vi "PicoScope3000aGetRapidBlockBulk.vi"(0 "error in":errorcluster, 5 "Number of Segments":u32, 7 "handle in":i16, 9 "Device Info":T1, 11 "Rapid Block Bulk Acquisition Settings":T2 {"Down Sample Ratio" min=1 step=1; "Down-Sample Mode" items=["None", "Aggregate", "Decimate", "Average"]}) -> (2 "Channel A Buffer":i16[][](array[numeric]), 3 "Channel B Buffer":i16[][](array[numeric]), 4 "error out":errorcluster, 6 "handle out":i16, 10 "Port 0 Buffer":i16[][](array[numeric]), 12 "Num samples":u32, 13 "Channel C Buffer":i16[][](array[numeric]), 14 "Channel D Buffer":i16[][](array[numeric]), 15 "Port 1 Buffer":i16[][](array[numeric]))   [LabVIEW 2009]
doc: "This VI gets a set of blocks captured using rapid block mode. It outputs two-dimensional arrays for each channel that contain data from all the requested captures."
uses:
  ps3000a.dll
panel:
  out "overflow":i16[](array[numeric])
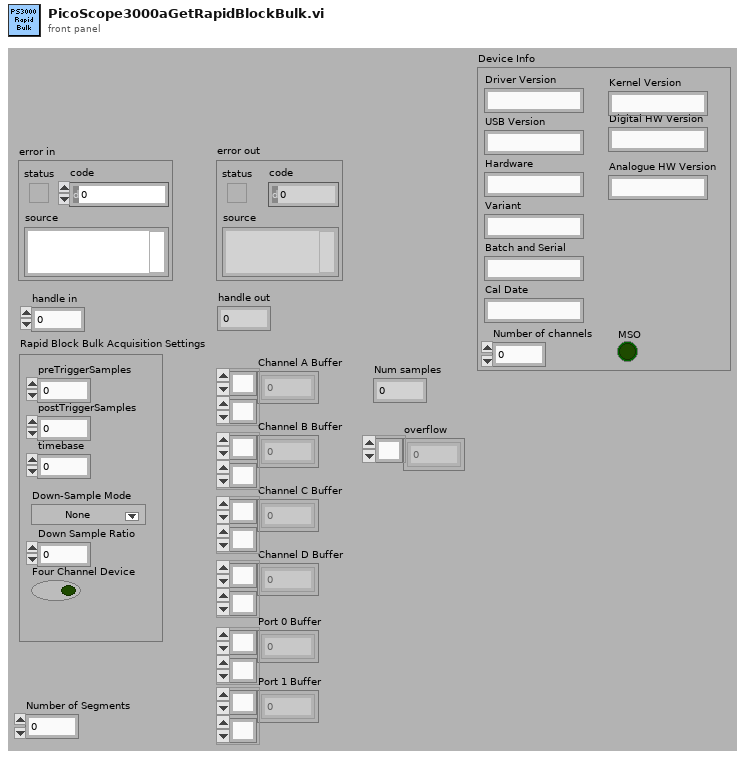
[diagram p1: front panel]
types:
  T1 = cluster{"Driver Version":string, "USB Version":string, "Hardware":string, "Variant":string, "Batch and Serial":string, "Cal Date":string, "Kernel Version":string, "Digital HW Version":string, "Analogue HW Version":string, "MSO":bool, "Number of channels":i16}
  T2 = cluster{"preTriggerSamples":u32, "postTriggerSamples":u32, "timebase":u32, "Down-Sample Mode":i32, "Down Sample Ratio":u32, "Four Channel Device":bool}
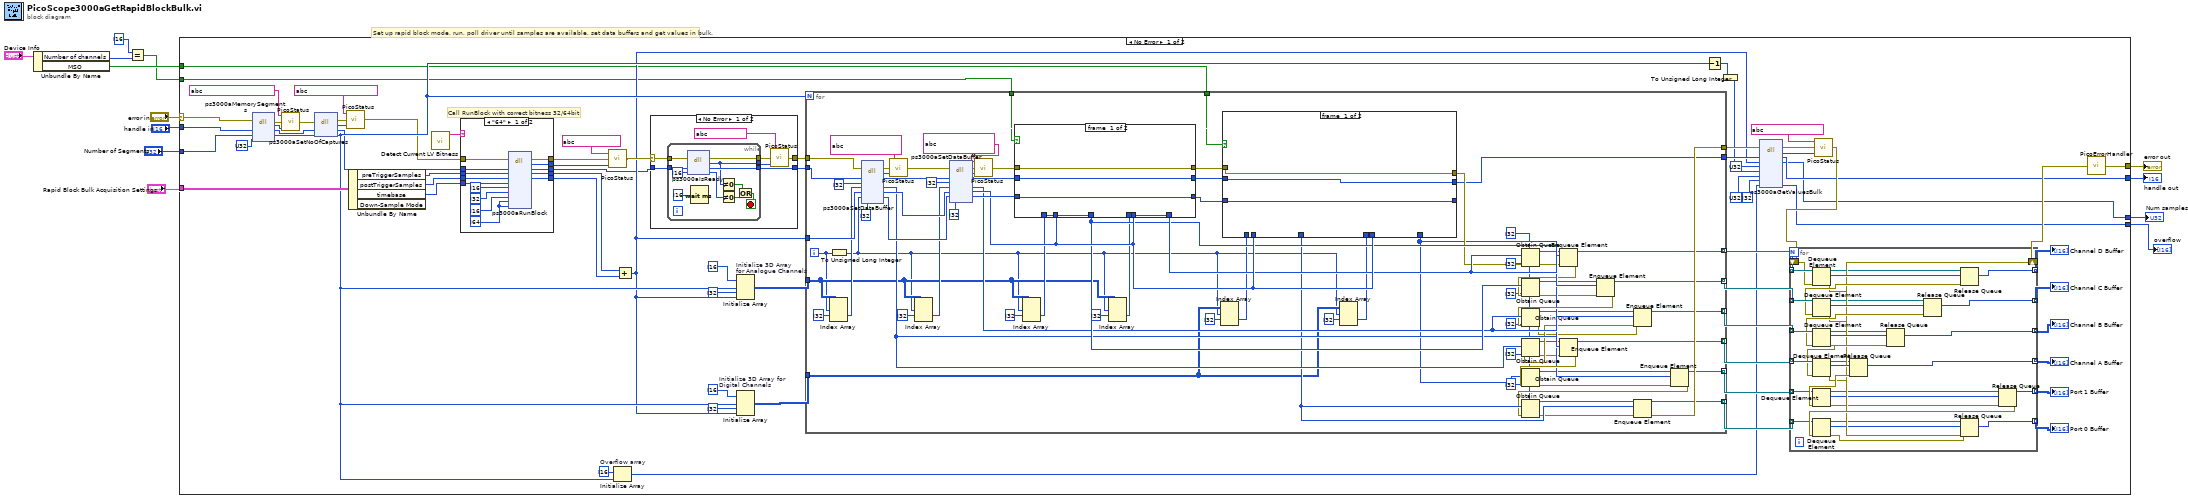
[diagram p0: block diagram]
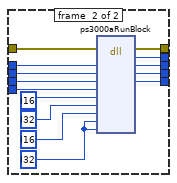
[diagram p2: hidden frame]
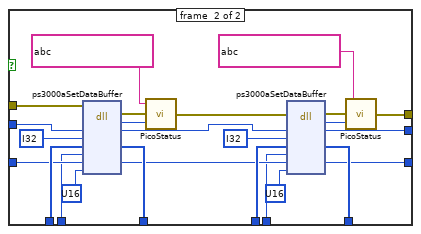
[diagram p3: hidden frame]
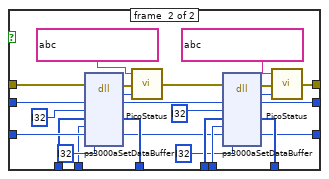
[diagram p4: hidden frame]
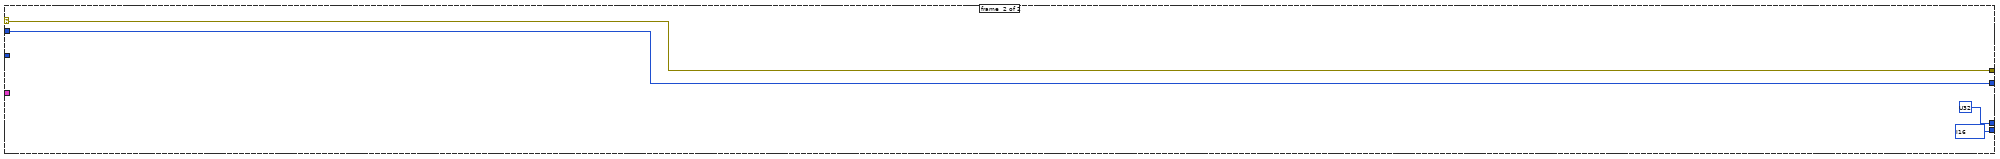
[diagram p6: hidden frame]
diagram:
  # "Set up rapid block mode, run, poll driver until samples are available, set data buffers and get values in bulk."
  n1 = Unbundle By Name("Device Info") -> ("Number of channels"=w4:i16, "MSO"=w5:bool)
  n2 = Equal?(x=i16 ?, y=w4) -> (x = y?=w2:bool)
  n3 = case shown="No Error" "error in" {
    selector: "error in" -> [w78 w303]
    tunnel: [w66 w303] -> w12
    tunnel: "handle in" -> [w77 w302]
    tunnel: [w56 w302] -> w10
    tunnel: [w31 u32 ?] -> w9
    tunnel: "Rapid Block Bulk Acquisition Settings" -> [w29 _]
    tunnel: "Number of Segments" -> [w28 _]
    tunnel: w2 -> [w26 _]
    tunnel: w5 -> [w27 _]
    tunnel: [w14 i16[] ? ("overflow")] -> w1
    frame #0 {
      # "Call RunBlock with correct bitness 32/64bit"
      n4 = dll-call lib="ps3000a.dll" fn="ps3000aMemorySegments" ("ps3000.dll:_ps3000_open_unit@0")(error in=w78, "handle"=w77, "nSegments"=w28, "nMaxSamples"=u32 ?) -> (error out=w75:errorcluster, "PICO_STATUS"=w76:i32, "handle"=w71:i16, "nSegments"=w72:u32)  [unwired: 3 in, 1 out]
      n5 = call "PicoStatus.vi"("PICO STATUS"=w76, "error in"=w75, "source"=string ?) -> ("error out"=w70:errorcluster)
      n6 = dll-call lib="ps3000a.dll" fn="ps3000aSetNoOfCaptures" ("ps3000.dll:_ps3000_open_unit@0")(error in=w70, "handle"=w71, "nCaptures"=w72) -> (error out=w68:errorcluster, "PICO_STATUS"=w69:i32, "handle"=w19:i16, "nCaptures"=w34:u32)  [unwired: 2 in, 1 out]
      n7 = call "PicoStatus.vi"("PICO STATUS"=w69, "error in"=w68, "source"=string ?) -> ("error out"=w15:errorcluster)
      n8 = Unbundle By Name(w29) -> ("preTriggerSamples"=w18:u32, "postTriggerSamples"=w17:u32, "timebase"=w16:u32)  [unwired: 1 out]
      n9 = call "Detect Current LV Bitness.vi"() -> ("bitness"=w25:string)  [unwired: 11 in]
      n10 = case shown="\"64\"" w25 {
        tunnel: [w96 w110] -> w22
        tunnel: [w95 w109] -> w21
        tunnel: [w94 w108] -> w20
        tunnel: w16 -> [w93 w107]
        tunnel: w18 -> [w92 w106]
        tunnel: w17 -> [w91 w105]
        tunnel: [w90 w104] -> w23
        tunnel: [w89 w103] -> w24
        tunnel: w15 -> [w88 w102]
        tunnel: w19 -> [w87 w101]
        frame #0 {
          w83 = i64 ? ("pParameter")
          n11 = dll-call lib="ps3000a.dll" fn="ps3000aRunBlock" ("ps3000.dll:_ps3000_open_unit@0")(error in=w88, "handle"=w87, "preTriggerSamples"=w92, "postTriggerSamples"=w91, "timebase"=w93, "oversample"=i16 ?, "timeindisposed"=i32 ? ("pParameter"), "segmentIndex"=i16 ? ("pParameter"), "lpReady"=w83, "pParameter"=w83) -> (error out=w89:errorcluster, "PICO_STATUS"=w90:i32, "handle"=w96:i16, "preTriggerSamples"=w95:u32, "postTriggerSamples"=w94:u32)  [unwired: 8 in, 1 out]
        }
        frame #1 {
          w97 = i32 ? ("pParameter")
          n12 = dll-call lib="ps3000a.dll" fn="ps3000aRunBlock" ("ps3000.dll:_ps3000_open_unit@0")(error in=w102, "handle"=w101, "preTriggerSamples"=w106, "postTriggerSamples"=w105, "timebase"=w107, "oversample"=i16 ?, "timeindisposed"=i32 ? ("pParameter"), "segmentIndex"=i16 ? ("pParameter"), "lpReady"=w97, "pParameter"=w97) -> (error out=w103:errorcluster, "PICO_STATUS"=w104:i32, "handle"=w110:i16, "preTriggerSamples"=w109:u32, "postTriggerSamples"=w108:u32)  [unwired: 8 in, 1 out]
        }
      }
      n13 = call "PicoStatus.vi"("PICO STATUS"=w23, "error in"=w24, "source"=string ?) -> ("error out"=w80:errorcluster)
      n14 = Initialize Array "Overflow array"(i16 ? ("element"), w34) -> (w40:i16[])
      n15 = Add(x=w21, y=w20) -> (x+y=w33:u32)
      n16 = case shown="No Error" w80 {
        selector: w80 -> [w284 w298]
        tunnel: w22 -> [w286 w299]
        tunnel: [w285 w299] -> w82
        tunnel: [w283 w298] -> w81
        frame #0 {
          n17 = while {
            tunnel: [w297] -> w285
            tunnel: w286 -> [w296]
            tunnel: [w291] -> w281
            tunnel: w284 -> [w290]
            tunnel: [w289] -> w282
            stop <- w295 stop-if-true
            n18 = dll-call lib="ps3000a.dll" fn="ps3000aIsReady" ("ps3000.dll:_ps3000_open_unit@0")(error in=w290, "handle"=w296, "ready"=i16 ?) -> (error out=w289:errorcluster, "status"=w291:i32, "handle"=w297:i16, "ready"=w292:i16)  [unwired: 2 in, 1 out]
            n19 = Wait (ms)(milliseconds to wait=i16 ? ("ready")) -> ()  [unwired: 1 out]
            n20 = Not Equal To 0?(x=w291) -> (x != 0?=w293:bool)
            n21 = Not Equal To 0?(x=w292) -> (x != 0?=w294:bool)
            n22 = Or(x=w293, y=w294) -> (x .or. y?=w295:bool)
          }
          n23 = call "PicoStatus.vi"("PICO STATUS"=w281, "error in"=w282, "source"=string ?) -> ("error out"=w283:errorcluster)
        }
        frame #1 {
        }
      }
      n24 = Initialize Array "Initialize 3D Array\nfor Analogue Channels"(i16 ? ("element"), w34, i32 ? ("dimension size"), w33) -> (w37:i16[][][])
      n25 = Initialize Array "Initialize 3D Array for \nDigital Channels"(i16 ? ("element"), w34, i32 ? ("dimension size"), w33) -> (w32:i16[][][])
      n26 = for {
        N: w34 -> [_]
        tunnel: w82 -> [w221]
        tunnel: w81 -> [w219]
        tunnel: w26 -> [w213]
        tunnel: w27 -> [w201]
        tunnel: [w185] -> w55
        tunnel: [w184] -> w54 mode=indexing
        tunnel: [w183] -> w53 mode=indexing
        tunnel: [w182] -> w52 mode=indexing
        tunnel: [w181] -> w51 mode=indexing
        tunnel: [w180] -> w50 mode=indexing
        tunnel: [w179] -> w49 mode=indexing
        tunnel: [w177] -> w43
        tunnel: w37 -> [w167]
        tunnel: w33 -> [w176]
        tunnel: w32 -> [w161]
        i -> [w162]
        n27 = Index Array(array=w167, index (dim 0)=w162, index (dim 1)=i32 ? ("disabled index (row)")) -> (element=w174:i16[])  [unwired: 1 in]
        n28 = To Unsigned Long Integer(number=w162) -> (unsigned 32bit integer=w160:u32)
        n29 = dll-call lib="ps3000a.dll" fn="ps3000aSetDataBuffer" ("ps3000.dll:_ps3000_open_unit@0")(error in=w219, "handle"=w221, "channel"=i32 ?, "buffer"=w174, "bufferLth"=w176, "waveform"=w160, "downSampleRatioMode"=i32 ?) -> (error out=w217:errorcluster, "PICO_STATUS"=w218:i32, "handle"=w209:i16, "buffer"=w193:i16[], "bufferLth"=w207:i32, "waveform"=w206:u32)  [unwired: 4 in, 1 out]
        n30 = call "PicoStatus.vi"("PICO STATUS"=w218, "error in"=w217, "source"=string ?) -> ("error out"=w210:errorcluster)
        n31 = Index Array(array=w167, index (dim 0)=w160, index (dim 1)=i32 ? ("disabled index (row)")) -> (element=w172:i16[])  [unwired: 1 in]
        n32 = dll-call lib="ps3000a.dll" fn="ps3000aSetDataBuffer" ("ps3000.dll:_ps3000_open_unit@0")(error in=w210, "handle"=w209, "channel"=i32 ?, "buffer"=w172, "bufferLth"=w207, "waveform"=w206, "downSampleRatioMode"=i32 ?) -> (error out=w212:errorcluster, "PICO_STATUS"=w211:i32, "handle"=w205:i16, "buffer"=w194:i16[], "bufferLth"=w197:i32, "waveform"=w204:u32)  [unwired: 4 in, 1 out]
        n33 = call "PicoStatus.vi"("PICO STATUS"=w211, "error in"=w212, "source"=string ?) -> ("error out"=w216:errorcluster)
        n34 = Index Array(array=w167, index (dim 0)=w160, index (dim 1)=i32 ? ("disabled index (row)")) -> (element=w170:i16[])  [unwired: 1 in]
        n35 = Index Array(array=w167, index (dim 0)=w160, index (dim 1)=i32 ? ("disabled index (row)")) -> (element=w168:i16[])  [unwired: 1 in]
        n36 = case shown="True" w213 {
          tunnel: w205 -> [w252 w270]
          tunnel: [w252 w264] -> w199
          tunnel: w170 -> [w254 w272]
          tunnel: w168 -> [w253 w260]
          tunnel: [w253 w266] -> w196
          tunnel: [w254 w274] -> w195
          tunnel: w216 -> [w251 w269]
          tunnel: [w251 w279] -> w200
          tunnel: w197 -> [_ w255]
          tunnel: w197 -> [_ w259]
          tunnel: w204 -> [w250 w273]
          tunnel: [w250 w265] -> w198
          frame #0 {
          }
          frame #1 {
            n37 = dll-call lib="ps3000a.dll" fn="ps3000aSetDataBuffer" ("ps3000.dll:_ps3000_open_unit@0")(error in=w269, "handle"=w270, "channel"=i32 ?, "buffer"=w272, "bufferLth"=w255, "waveform"=w273, "downSampleRatioMode"=i32 ?) -> (error out=w276:errorcluster, "PICO_STATUS"=w275:i32, "handle"=w263:i16, "buffer"=w274:i16[], "waveform"=w258:u32)  [unwired: 5 in, 1 out]
            n38 = call "PicoStatus.vi"("PICO STATUS"=w275, "error in"=w276, "source"=string ?) -> ("error out"=w262:errorcluster)
            n39 = dll-call lib="ps3000a.dll" fn="ps3000aSetDataBuffer" ("ps3000.dll:_ps3000_open_unit@0")(error in=w262, "handle"=w263, "channel"=i32 ?, "buffer"=w260, "bufferLth"=w259, "waveform"=w258, "downSampleRatioMode"=i32 ?) -> (error out=w268:errorcluster, "PICO_STATUS"=w267:i32, "handle"=w264:i16, "buffer"=w266:i16[], "waveform"=w265:u32)  [unwired: 5 in, 1 out]
            n40 = call "PicoStatus.vi"("PICO STATUS"=w267, "error in"=w268, "source"=string ?) -> ("error out"=w279:errorcluster)
          }
        }
        n41 = Index Array(array=w161, index (dim 0)=w160, index (dim 1)=i32 ? ("disabled index (row)")) -> (element=w165:i16[])  [unwired: 1 in]
        n42 = Index Array(array=w161, index (dim 0)=w160, index (dim 1)=i32 ? ("disabled index (row)")) -> (element=w163:i16[])  [unwired: 1 in]
        n43 = case shown="True" w201 {
          tunnel: w200 -> [w224 w249]
          tunnel: w199 -> [w223 w248]
          tunnel: w165 -> [_ w246]
          tunnel: w197 -> [_ w226]
          tunnel: w163 -> [_ w244]
          tunnel: [_ w243] -> w192
          tunnel: [_ w242] -> w178
          tunnel: [w223 w236] -> w177
          tunnel: [w224 w235] -> w191
          tunnel: w198 -> [w222 w230]
          tunnel: w197 -> [_ w228]
          tunnel: [w222 w225] -> _
          frame #0 {
          }
          frame #1 {
            n44 = dll-call lib="ps3000a.dll" fn="ps3000aSetDataBuffer" ("ps3000.dll:_ps3000_open_unit@0")(error in=w249, "handle"=w248, "channel"=i32 ?, "buffer"=w246, "bufferLth"=w228, "segmentIndex"=w230, "mode"=u16 ? ("segmentIndex")) -> (error out=w240:errorcluster, "PICO_STATUS"=w241:i32, "handle"=w234:i16, "buffer"=w243:i16[], "segmentIndex"=w229:u32)  [unwired: 5 in, 1 out]
            n45 = call "PicoStatus.vi"("PICO STATUS"=w241, "error in"=w240, "source"=string ?) -> ("error out"=w237:errorcluster)
            n46 = dll-call lib="ps3000a.dll" fn="ps3000aSetDataBuffer" ("ps3000.dll:_ps3000_open_unit@0")(error in=w237, "handle"=w234, "channel"=i32 ?, "buffer"=w244, "bufferLth"=w226, "segmentIndex"=w229, "mode"=u16 ? ("segmentIndex")) -> (error out=w238:errorcluster, "PICO_STATUS"=w239:i32, "handle"=w236:i16, "buffer"=w242:i16[], "segmentIndex"=w225:u32)  [unwired: 5 in, 1 out]
            n47 = call "PicoStatus.vi"("PICO STATUS"=w239, "error in"=w238, "source"=string ?) -> ("error out"=w235:errorcluster)
          }
        }
        n48 = Obtain Queue(max queue size (-1, unlimited)=i32 ?, element data type=w196, error in (no error)=w191) -> (queue out=w145:refnum<queue>, error out=w146:errorcluster)  [unwired: 2 in, 1 out]
        n49 = Enqueue Element(queue=w145, element=w196, error in (no error)=w146) -> (queue out=w184:refnum<queue>, error out=w190:errorcluster)  [unwired: 1 in, 1 out]
        n50 = Obtain Queue(max queue size (-1, unlimited)=i32 ?, element data type=w195, error in (no error)=w190) -> (queue out=w148:refnum<queue>, error out=w149:errorcluster)  [unwired: 2 in, 1 out]
        n51 = Enqueue Element(queue=w148, element=w195, error in (no error)=w149) -> (queue out=w183:refnum<queue>, error out=w189:errorcluster)  [unwired: 1 in, 1 out]
        n52 = Obtain Queue(max queue size (-1, unlimited)=i32 ?, element data type=w194, error in (no error)=w189) -> (queue out=w151:refnum<queue>, error out=w152:errorcluster)  [unwired: 2 in, 1 out]
        n53 = Enqueue Element(queue=w151, element=w194, error in (no error)=w152) -> (queue out=w182:refnum<queue>, error out=w188:errorcluster)  [unwired: 1 in, 1 out]
        n54 = Obtain Queue(max queue size (-1, unlimited)=i32 ?, element data type=w193, error in (no error)=w188) -> (queue out=w142:refnum<queue>, error out=w143:errorcluster)  [unwired: 2 in, 1 out]
        n55 = Enqueue Element(queue=w142, element=w193, error in (no error)=w143) -> (queue out=w181:refnum<queue>, error out=w187:errorcluster)  [unwired: 1 in, 1 out]
        n56 = Obtain Queue(max queue size (-1, unlimited)=i32 ?, element data type=w178, error in (no error)=w187) -> (queue out=w157:refnum<queue>, error out=w158:errorcluster)  [unwired: 2 in, 1 out]
        n57 = Enqueue Element(queue=w157, element=w178, error in (no error)=w158) -> (queue out=w180:refnum<queue>, error out=w186:errorcluster)  [unwired: 1 in, 1 out]
        n58 = Obtain Queue(max queue size (-1, unlimited)=i32 ?, element data type=w192, error in (no error)=w186) -> (queue out=w154:refnum<queue>, error out=w155:errorcluster)  [unwired: 2 in, 1 out]
        n59 = Enqueue Element(queue=w154, element=w192, error in (no error)=w155) -> (queue out=w179:refnum<queue>, error out=w185:errorcluster)  [unwired: 1 in, 1 out]
      }
      n60 = Decrement(x=w34) -> (x-1=w42:u32)
      n61 = To Unsigned Long Integer(number=w42) -> (unsigned 32bit integer=w30:u32)
      n62 = dll-call lib="ps3000a.dll" fn="ps3000aGetValuesBulk" ("ps3000.dll:_ps3000_open_unit@0")(error in=w55, "handle"=w43, "noOfSamples"=w33, "fromSegmentIndex"=u32 ?, "toSegmentIndex"=w30, "downSampleRatio"=u32 ?, "downSampleRatioMode"=i32 ?, "overflow"=w40) -> (error out=w59:errorcluster, "PICO_STATUS"=w58:i32, "handle"=w56:i16, "noOfSamples"=w31:u32, "overflow"=w14:i16[])  [unwired: 6 in, 1 out]
      n63 = call "PicoStatus.vi"("PICO STATUS"=w58, "error in"=w59, "source"=string ?) -> ("error out"=w57:errorcluster)
      n64 = for {
        tunnel: w51 -> [w141] mode=indexing
        tunnel: [w140] -> w60 mode=indexing
        shift-right: [w127] -> w64
        shift-left: w57 -> [w136]
        tunnel: w52 -> [w139] mode=indexing
        tunnel: w54 -> [w138] mode=indexing
        tunnel: w53 -> [w137] mode=indexing
        tunnel: [w132] -> w63 mode=indexing
        tunnel: [w131] -> w62 mode=indexing
        tunnel: [w130] -> w61 mode=indexing
        tunnel: w50 -> [w126] mode=indexing
        tunnel: w49 -> [w125] mode=indexing
        tunnel: [w124] -> w48 mode=indexing
        tunnel: [w123] -> w47 mode=indexing
        n65 = Dequeue Element(queue=w138, error in (no error)=w136) -> (queue out=w118:refnum<queue>, element=w132:i16[], error out=w117:errorcluster)  [unwired: 1 in, 1 out]
        n66 = Release Queue(queue=w118, error in (no error)=w117) -> (error out=w135:errorcluster)  [unwired: 1 in, 2 out]
        n67 = Dequeue Element(queue=w137, error in (no error)=w135) -> (queue out=w116:refnum<queue>, element=w131:i16[], error out=w115:errorcluster)  [unwired: 1 in, 1 out]
        n68 = Release Queue(queue=w116, error in (no error)=w115) -> (error out=w134:errorcluster)  [unwired: 1 in, 2 out]
        n69 = Dequeue Element(queue=w139, error in (no error)=w134) -> (queue out=w114:refnum<queue>, element=w130:i16[], error out=w113:errorcluster)  [unwired: 1 in, 1 out]
        n70 = Release Queue(queue=w114, error in (no error)=w113) -> (error out=w133:errorcluster)  [unwired: 1 in, 2 out]
        n71 = Dequeue Element(queue=w141, error in (no error)=w133) -> (queue out=w112:refnum<queue>, element=w140:i16[], error out=w111:errorcluster)  [unwired: 1 in, 1 out]
        n72 = Release Queue(queue=w112, error in (no error)=w111) -> (error out=w129:errorcluster)  [unwired: 1 in, 2 out]
        n73 = Dequeue Element(queue=w126, error in (no error)=w129) -> (queue out=w122:refnum<queue>, element=w124:i16[], error out=w121:errorcluster)  [unwired: 1 in, 1 out]
        n74 = Release Queue(queue=w122, error in (no error)=w121) -> (error out=w128:errorcluster)  [unwired: 1 in, 2 out]
        n75 = Dequeue Element(queue=w125, error in (no error)=w128) -> (queue out=w120:refnum<queue>, element=w123:i16[], error out=w119:errorcluster)  [unwired: 1 in, 1 out]
        n76 = Release Queue(queue=w120, error in (no error)=w119) -> (error out=w127:errorcluster)  [unwired: 1 in, 2 out]
      }
      "Channel D Buffer" <- w63
      "Channel C Buffer" <- w62
      "Channel B Buffer" <- w61
      "Channel A Buffer" <- w60
      "Port 0 Buffer" <- w47
      "Port 1 Buffer" <- w48
      n77 = call "PicoErrorHandler.vi"("error in"=w64) -> ("error out"=w66:errorcluster)
    }
    frame #1 {
    }
  }
  "error out" <- w12
  "handle out" <- w10
  "Num samples" <- w9
  "overflow" <- w1
